vi "Create Room.vi"(8 "error in":errorcluster, 9 "State":bool[](array[boolean])=[FALSE, FALSE, FALSE, FALSE], 10 "Color":T1[](array[typedef])=[enum."Red", enum."Blue", enum."Green", enum."Yellow"], 11 "Room Number":u32) -> (0 "error out":errorcluster, 3 "Room Ref":refnum<class "Room.lvclass">)   [LabVIEW 2015, in "Room.lvclass"]
uses:
  Room.lvclass
  Flags/ColorEnum.ctl
  Room.lvclass/Room.ctl
  Write Flags.lvclass.vi
  Write BedVacant.vi
  Write InRoomPersonnel.vi
  Write RoomRequests.vi
  Flags/Flags.lvclass
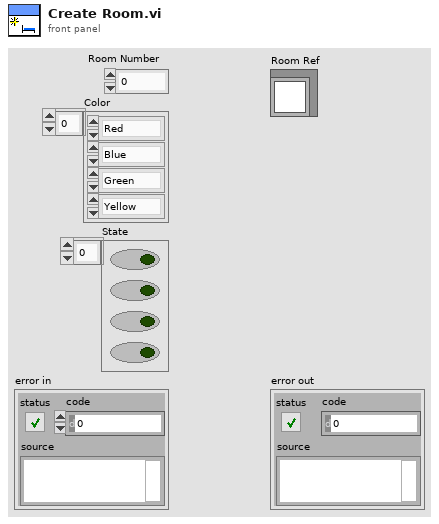
[diagram p1: front panel]
types:
  T1 = typedef "Flags.lvclass/ColorEnum.ctl" = enum8{"Red", "Blue", "Green", "Yellow"}
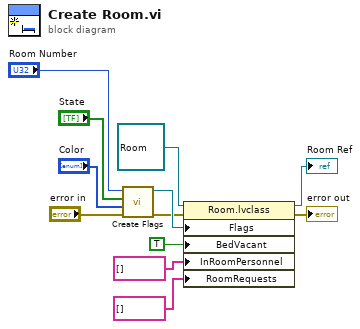
[diagram p0: block diagram]
diagram:
  n1 = call "Create Flags.vi"("error in"="error in", "Color"="Color", "State"="State", "Room Number"="Room Number") -> ("error out"=w10:errorcluster, "reference out"=w11:refnum<class "Flags.lvclass">)  [unwired: 6 in]
  n2 = property class="Room.lvclass"(reference=refnum<class "Room.lvclass"> refnum ("Room.lvclass"), error in=w10, "Flags"=w11, "BedVacant"=TRUE, "InRoomPersonnel"=string[] [], "RoomRequests"=string[] []) -> (reference out=→"Room Ref":refnum<class "Room.lvclass">, error out=→"error out":errorcluster)
